vi "1B Simulator Initializer.vi"(10 "Simulator\nBounds":T1={"Simulator E Range"=20.0, "Simulator E Min"=-10.0, "Simulator N Range"=20.0, "Simulator N Min"=-10.0}) -> ()   [LabVIEW 2011]
doc: "An initialization routine for the simulator. Resets all relevant characteristiscs (rate of turn, heading, velocity), places simulated boat in center of map, and creates no sail zones around the edges of the map."
uses:
  2-Think/2 Typedefs/rate of turn.ctl
  2-Think/2 Typedefs/heading.ctl
  2-Think/2 Typedefs/robot velocity.ctl
  2-Think/2 Typedefs/UTM Location.ctl
  2-Think/2 Globals/2 Global.vi
  2-Think/2 Typedefs/UTM Circle.ctl
  1,3 B Typedefs/simulator bounds.ctl
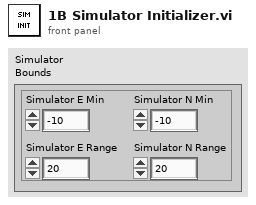
[diagram p1: front panel]
types:
  T1 = typedef "simulator bounds.ctl" = cluster{"Simulator E Range":dbl, "Simulator E Min":dbl, "Simulator N Range":dbl, "Simulator N Min":dbl}
  T2 = typedef "UTM Location.ctl" = cluster{"UTM Zone":dbl, "Hemisphere":enum16{"North", "South"}, "East":dbl, "North":dbl}
  T3 = typedef "robot velocity.ctl" = cluster{"East":dbl, "North":dbl}
  T4 = typedef "heading.ctl" = dbl
  T5 = typedef "rate of turn.ctl" = dbl
  T6 = typedef "UTM Circle.ctl" = cluster{"UTM Zone":dbl, "Hemisphere":enum16{"North", "South"}, "East":dbl, "North":dbl, "Radius":dbl}
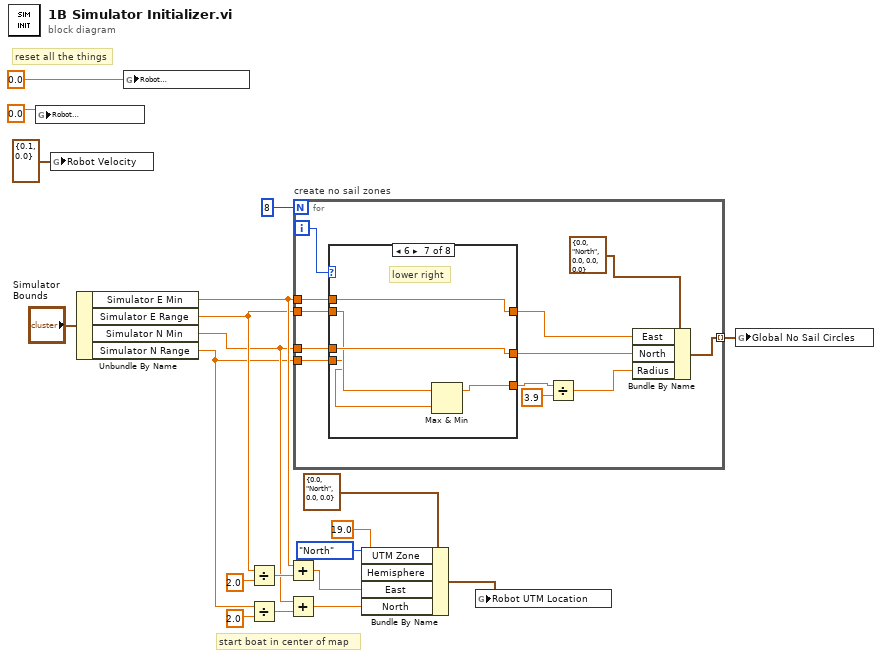
[diagram p0: block diagram]
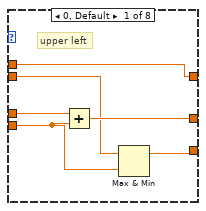
[diagram p2: hidden frame]
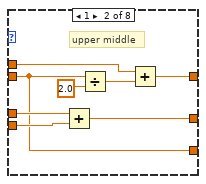
[diagram p3: hidden frame]
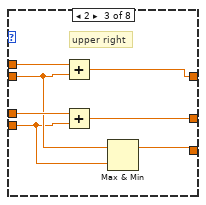
[diagram p4: hidden frame]
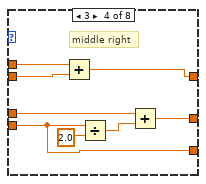
[diagram p5: hidden frame]
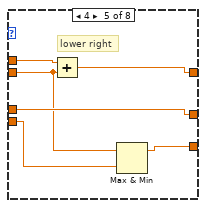
[diagram p6: hidden frame]
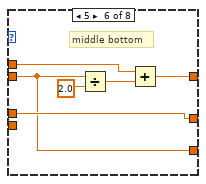
[diagram p7: hidden frame]
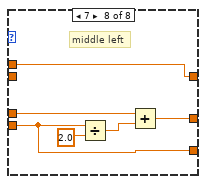
[diagram p8: hidden frame]
diagram:
  # "start boat in center of map"
  # "reset all the things"
  n1 = global write "2 Global.vi" "Robot\nHeading"(T4 0.0 ("Robot\nHeading")) -> ()
  n2 = global write "2 Global.vi" "Robot Velocity"(T3 {"East"=0.1, "North"=0.0} ("Robot Velocity")) -> ()
  n3 = Unbundle By Name("Simulator\nBounds") -> ("Simulator E Min"=w7:dbl, "Simulator E Range"=w6:dbl, "Simulator N Min"=w5:dbl, "Simulator N Range"=w4:dbl)
  n4 = global write "2 Global.vi" "Robot\nRate of Turn"(T5 0.0 ("Robot\nRate of Turn")) -> ()
  n5 = Divide(x=w6, y=2.0) -> (x/y=w11:dbl)
  n6 = Divide(x=w4, y=2.0) -> (x/y=w9:dbl)
  n7 = Add(x=w7, y=w11) -> (x+y=w15:dbl)
  n8 = Add(x=w5, y=w9) -> (x+y=w14:dbl)
  n9 = for "create no sail zones" {
    N: 8 -> [_]
    tunnel: w7 -> [w31]
    tunnel: w6 -> [w27]
    tunnel: w5 -> [w29]
    tunnel: w4 -> [w26]
    tunnel: [w23] -> w3 mode=indexing
    i -> [w22]
    n10 = case shown="6" w22 {
      tunnel: w31 -> [w36 w45 w51 w58 w66 w71 w78 w84]
      tunnel: [w36 w46 w50 w59 w67 w73 w78 w84] -> w30
      tunnel: w29 -> [w38 w41 w52 w60 w65 w69 w77 w80]
      tunnel: [w37 w40 w53 w61 w65 w69 w77 w83] -> w28
      tunnel: w26 -> [w33 w42 w47 w54 w63 _ w74 w79]
      tunnel: w27 -> [w34 w39 w48 w57 w62 w68 w75 _]
      tunnel: [w35 w39 w49 w54 w64 w68 w76 w79] -> w21
      frame 0, Default {
        # "upper left"
        n11 = Add(x=w38, y=w33) -> (x+y=w37:dbl)
        n12 = Max & Min(x=w34, y=w33) -> (max(x,y)=w35:dbl)  [unwired: 1 out]
      }
      frame 1 {
        # "upper middle"
        n13 = Add(x=w41, y=w42) -> (x+y=w40:dbl)
        n14 = Divide(x=w39, y=2.0) -> (x/y=w44:dbl)
        n15 = Add(x=w45, y=w44) -> (x+y=w46:dbl)
      }
      frame 2 {
        # "upper right"
        n16 = Add(x=w51, y=w48) -> (x+y=w50:dbl)
        n17 = Add(x=w52, y=w47) -> (x+y=w53:dbl)
        n18 = Max & Min(x=w48, y=w47) -> (max(x,y)=w49:dbl)  [unwired: 1 out]
      }
      frame 3 {
        # "middle right"
        n19 = Add(x=w58, y=w57) -> (x+y=w59:dbl)
        n20 = Divide(x=w54, y=2.0) -> (x/y=w56:dbl)
        n21 = Add(x=w60, y=w56) -> (x+y=w61:dbl)
      }
      frame 4 {
        # "lower right"
        n22 = Add(x=w66, y=w62) -> (x+y=w67:dbl)
        n23 = Max & Min(x=w62, y=w63) -> (max(x,y)=w64:dbl)  [unwired: 1 out]
      }
      frame 5 {
        # "middle bottom"
        n24 = Divide(x=w68, y=2.0) -> (x/y=w72:dbl)
        n25 = Add(x=w71, y=w72) -> (x+y=w73:dbl)
      }
      frame 6 {
        # "lower right"
        n26 = Max & Min(x=w75, y=w74) -> (max(x,y)=w76:dbl)  [unwired: 1 out]
      }
      frame 7 {
        # "middle left"
        n27 = Divide(x=w79, y=2.0) -> (x/y=w82:dbl)
        n28 = Add(x=w80, y=w82) -> (x+y=w83:dbl)
      }
    }
    n29 = Divide(x=w21, y=3.9) -> (x/y=w24:dbl)
    n30 = Bundle By Name(cluster=T6 {"UTM Zone"=0.0, "Hemisphere"=enum."North", "East"=0.0, "North"=0.0, "Radius"=0.0} ("UTM Location"), "East"=w30, "North"=w28, "Radius"=w24) -> (w23:T6)
  }
  n31 = Bundle By Name(cluster=T2 {"UTM Zone"=0.0, "Hemisphere"=enum."North", "East"=0.0, "North"=0.0} ("Robot UTM Location"), "UTM Zone"=19.0, "Hemisphere"=enum16{"North", "South"}."North", "East"=w15, "North"=w14) -> (w17:T2)
  n32 = global write "2 Global.vi" "Robot UTM Location"(w17) -> ()
  n33 = global write "2 Global.vi" "Global No Sail Circles"(w3) -> ()
